vi "final.vi"() -> ()   [LabVIEW 2020]
uses:
  <vilib>/Simulation/Scripting/Companion Diagram/SimConfigNode/SimParams.ctl
  <vilib>/Simulation/Scripting/Companion Diagram/SimConfigNode/_simSolvers.ctl
  <vilib>/Simulation/Implementation/Shared/SIMSCR Execution Mode.ctl
  <vilib>/Simulation/Param Hierarchy/Typedefs/SIMPH Param Control Actions.ctl
  <vilib>/Simulation/Implementation/Shared/SIM limit type.ctl
  <vilib>/Simulation/Implementation/Shared/NILVSim_ParamChanged.vi
  <vilib>/Simulation/Implementation/Shared/NILVSIM_BeginStep.vi
  <vilib>/Simulation/SignalArithmetic/Implementation/NILVSim Gain.llb/SIM Gain (scalar).vi
  <vilib>/Simulation/ContinuousLinear/Implementation/NILVSim Derivative.llb/SIM derivative (scalar).vi
  <vilib>/Simulation/SignalDisplay/Implementation/NILVSim Time Waveform.llb/SIM Time Waveform (vector).vi
  <vilib>/Simulation/ContinuousLinear/Implementation/NILVSim Integrator new.llb/SIM Integrator distributor (scalar).vi
  <vilib>/Simulation/ContinuousLinear/Implementation/NILVSim Integrator new.llb/SIM Integrator collector (scalar).vi
  <vilib>/Simulation/SignalDisplay/Implementation/NILVSim Time Waveform.llb/SIM Time Waveform (scalar).vi
  <vilib>/Simulation/Implementation/Shared/SIM Is Init or Final Stage.vi
  <vilib>/Simulation/Implementation/Shared/NILVSim_Manager.vi
  <vilib>/Utility/error.llb/Clear Errors.vi
  <vilib>/Simulation/Implementation/Shared/NILVSim_FinalizeModel.vi
  <vilib>/imath/engines/lvmath2/RunTimeEngine/Managers/WorkSpace/UID Generator.vi
  <vilib>/imath/engines/lvmath2/RunTimeEngine/RunTimeType/NIMS_RunTimeType_From StrictType (excl LVString).vi
  <instcachedir>/0/NIMS_RunTimeType_From StrictType (excl LVString)_283B1B2000484AAA8744D21CE97EA49F.lvgen/NIMS_RunTimeType_From StrictType (excl LVString)_283B1B2000484AAA8744D21CE97EA49F_000.vi
  <vilib>/imath/engines/lvmath2/RunTimeEngine/LocalVariableDefStatement/MC_LocalVariableDefStatement_Display.vi
  <vilib>/imath/engines/lvmath/Plug In/Control Design/BuiltInFunctions/tf/NIMS_CD_tf(num,den,Ts).vi
  <instcachedir>/0/NIMS_RunTimeType_From StrictType (excl LVString)_283B1B2000484AAA8744D21CE97EA49F.lvgen/NIMS_RunTimeType_From StrictType (excl LVString)_283B1B2000484AAA8744D21CE97EA49F_031.vi
  <vilib>/imath/engines/lvmath/Plug In/Control Design/BuiltInFunctions/series/NIMS_CD_series(TF,TF).vi
  <vilib>/imath/engines/lvmath/Plug In/Control Design/BuiltInFunctions/feedback/NIMS_CD_feedback(TF,K,SIGN).vi
  <vilib>/imath/engines/lvmath/Plug In/Control Design/BuiltInFunctions/poles/NIMS_CD_poles(TF).vi
  <vilib>/imath/engines/lvmath2/RunTimeEngine/Managers/SymbolTable/Clear UID.vi
  <vilib>/imath/engines/lvmath2/RunTimeEngine/NodeEndStatement/NIMS_NodeEndStatement_Output.vi
  <instcachedir>/0/NIMS_NodeEndStatement_Output_53EC0D466D134D7ABD903AC30B43404B.lvgen/NIMS_NodeEndStatement_Output_53EC0D466D134D7ABD903AC30B43404B_000.vi
  <instcachedir>/0/NIMS_NodeEndStatement_Output_53EC0D466D134D7ABD903AC30B43404B.lvgen/NIMS_NodeEndStatement_Output_53EC0D466D134D7ABD903AC30B43404B_010.vi
  <vilib>/imath/engines/lvmath2/RunTimeEngine/ErrorHandling/NIMS_Finalize Error.vi
  <vilib>/addons/Control Design/_Utility/Model Viewer.llb/Model Viewer SubVI/cd_Draw Transfer Function Equation (TF).vi
  <vilib>/Simulation/Implementation/Shared/SIM Unbundle Sim Info.vi
  <vilib>/Simulation/Implementation/Shared/NILVSim_Initialize.vi
  <vilib>/Simulation/Utility/Implementation/NILVSim Get Time and IsAcceptedStep.vi
  <vilib>/Platform/system.llb/Beep.vi
  <vilib>/Simulation/Implementation/Shared/SIMSH Read Queue.vi
  <vilib>/Simulation/Implementation/Shared/NILVSim_GetModelError.vi
  <vilib>/Simulation/Implementation/Shared/SIM Bundle Sim Info.vi
  <vilib>/Simulation/Scripting/Companion Diagram/SimConfigNode/SimDog.xnode
  <vilib>/Simulation/Implementation/XNodeFramework/SimXNode/SimX.xnode
  <vilib>/Simulation/ContinuousLinear/Implementation/NILVSim Integrator new.llb/SIM Integrator (scalar).vi
  <vilib>/addons/Control Design/_Utility/NI_CD_Model Viewer.lvlib
  <vilib>/imath/engines/lvmath2/RunTimeEngine/Managers/SymbolTable/NIMS_WorkSpace.lvlib
  <vilib>/Simulation/Implementation/Shared/NI_SIM_Implementation.lvlib
panel:
  out "Pososto sfalmatos peiramatikhs apo thewrtikh%":dbl format="%#_3g"
  out "Torque":waveform(dbl)(graph)
  out "Live gwniakh ta/xta":dynamicdata(graph)
  out "Gnwiakh ta/xta live":dbl
  out "Vout live":dbl
  out "p":cdb[](array[numeric])
  out "Gclosed with PID":picture
  out "PID open":picture
  out "Vout":dbl
  out "Current":dbl
  out "Gwniakh tax/ta":dbl
  in  "Vin":dbl
  out "Vout/Vin":waveform(dbl)[](graph)
  in  "Ki":dbl
  in  "Kd":dbl
  in  "Kp":dbl
  in  "R":dbl
  in  "b":dbl
  in  "L":dbl
  in  "J":dbl
  in  "K":dbl
  out "Gopen-DC Motor":picture
  out "Гщнйбкз фбч/фб":waveform(dbl)(graph)
  out "Current":waveform(dbl)(graph)
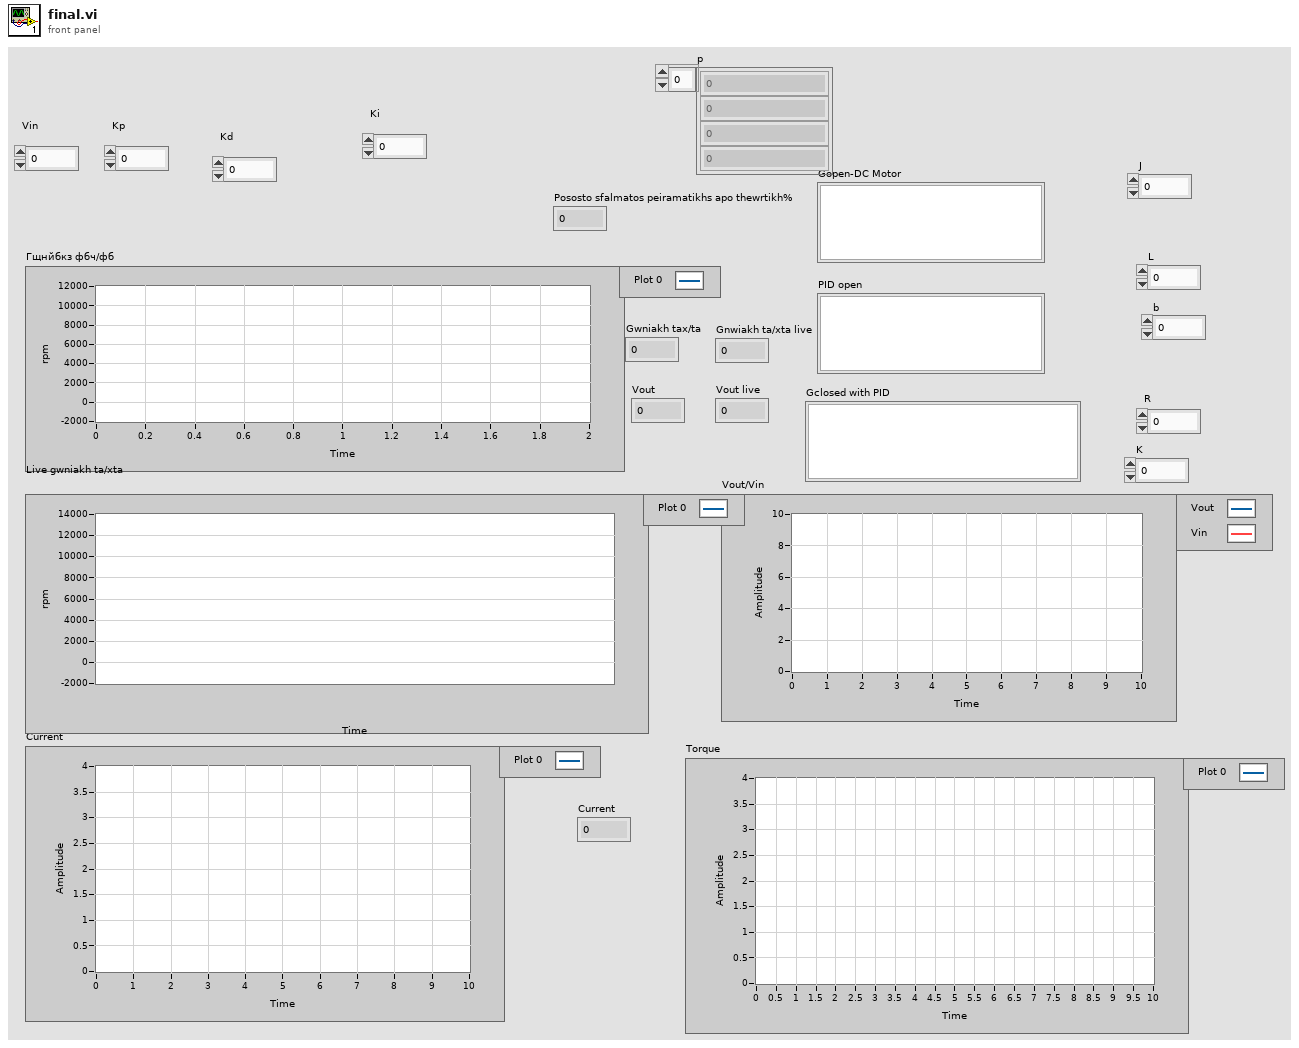
[diagram p1: front panel]
types:
  T1 = typedef "NI_LinSys_Model Typedefs.lvlib/CD Transfer Function Model (MIMO).ctl" = cluster{"properties":T2, "transfer function(s)":T3[][]}
  T2 = typedef "NI_LinSys_Model Typedefs.lvlib/CD General Elements.ctl" = cluster{"Model name":string, "Input names":string[], "Output names":string[], "Input Delays":dbl[], "Output Delays":dbl[], "Sampling Time":dbl, "Notes":string}
  T3 = typedef "NI_LinSys_Model Typedefs.lvlib/CD Transfer Function Model (SISO).ctl" = cluster{"Numerator":dbl[], "Denominator":dbl[], "delay":dbl}
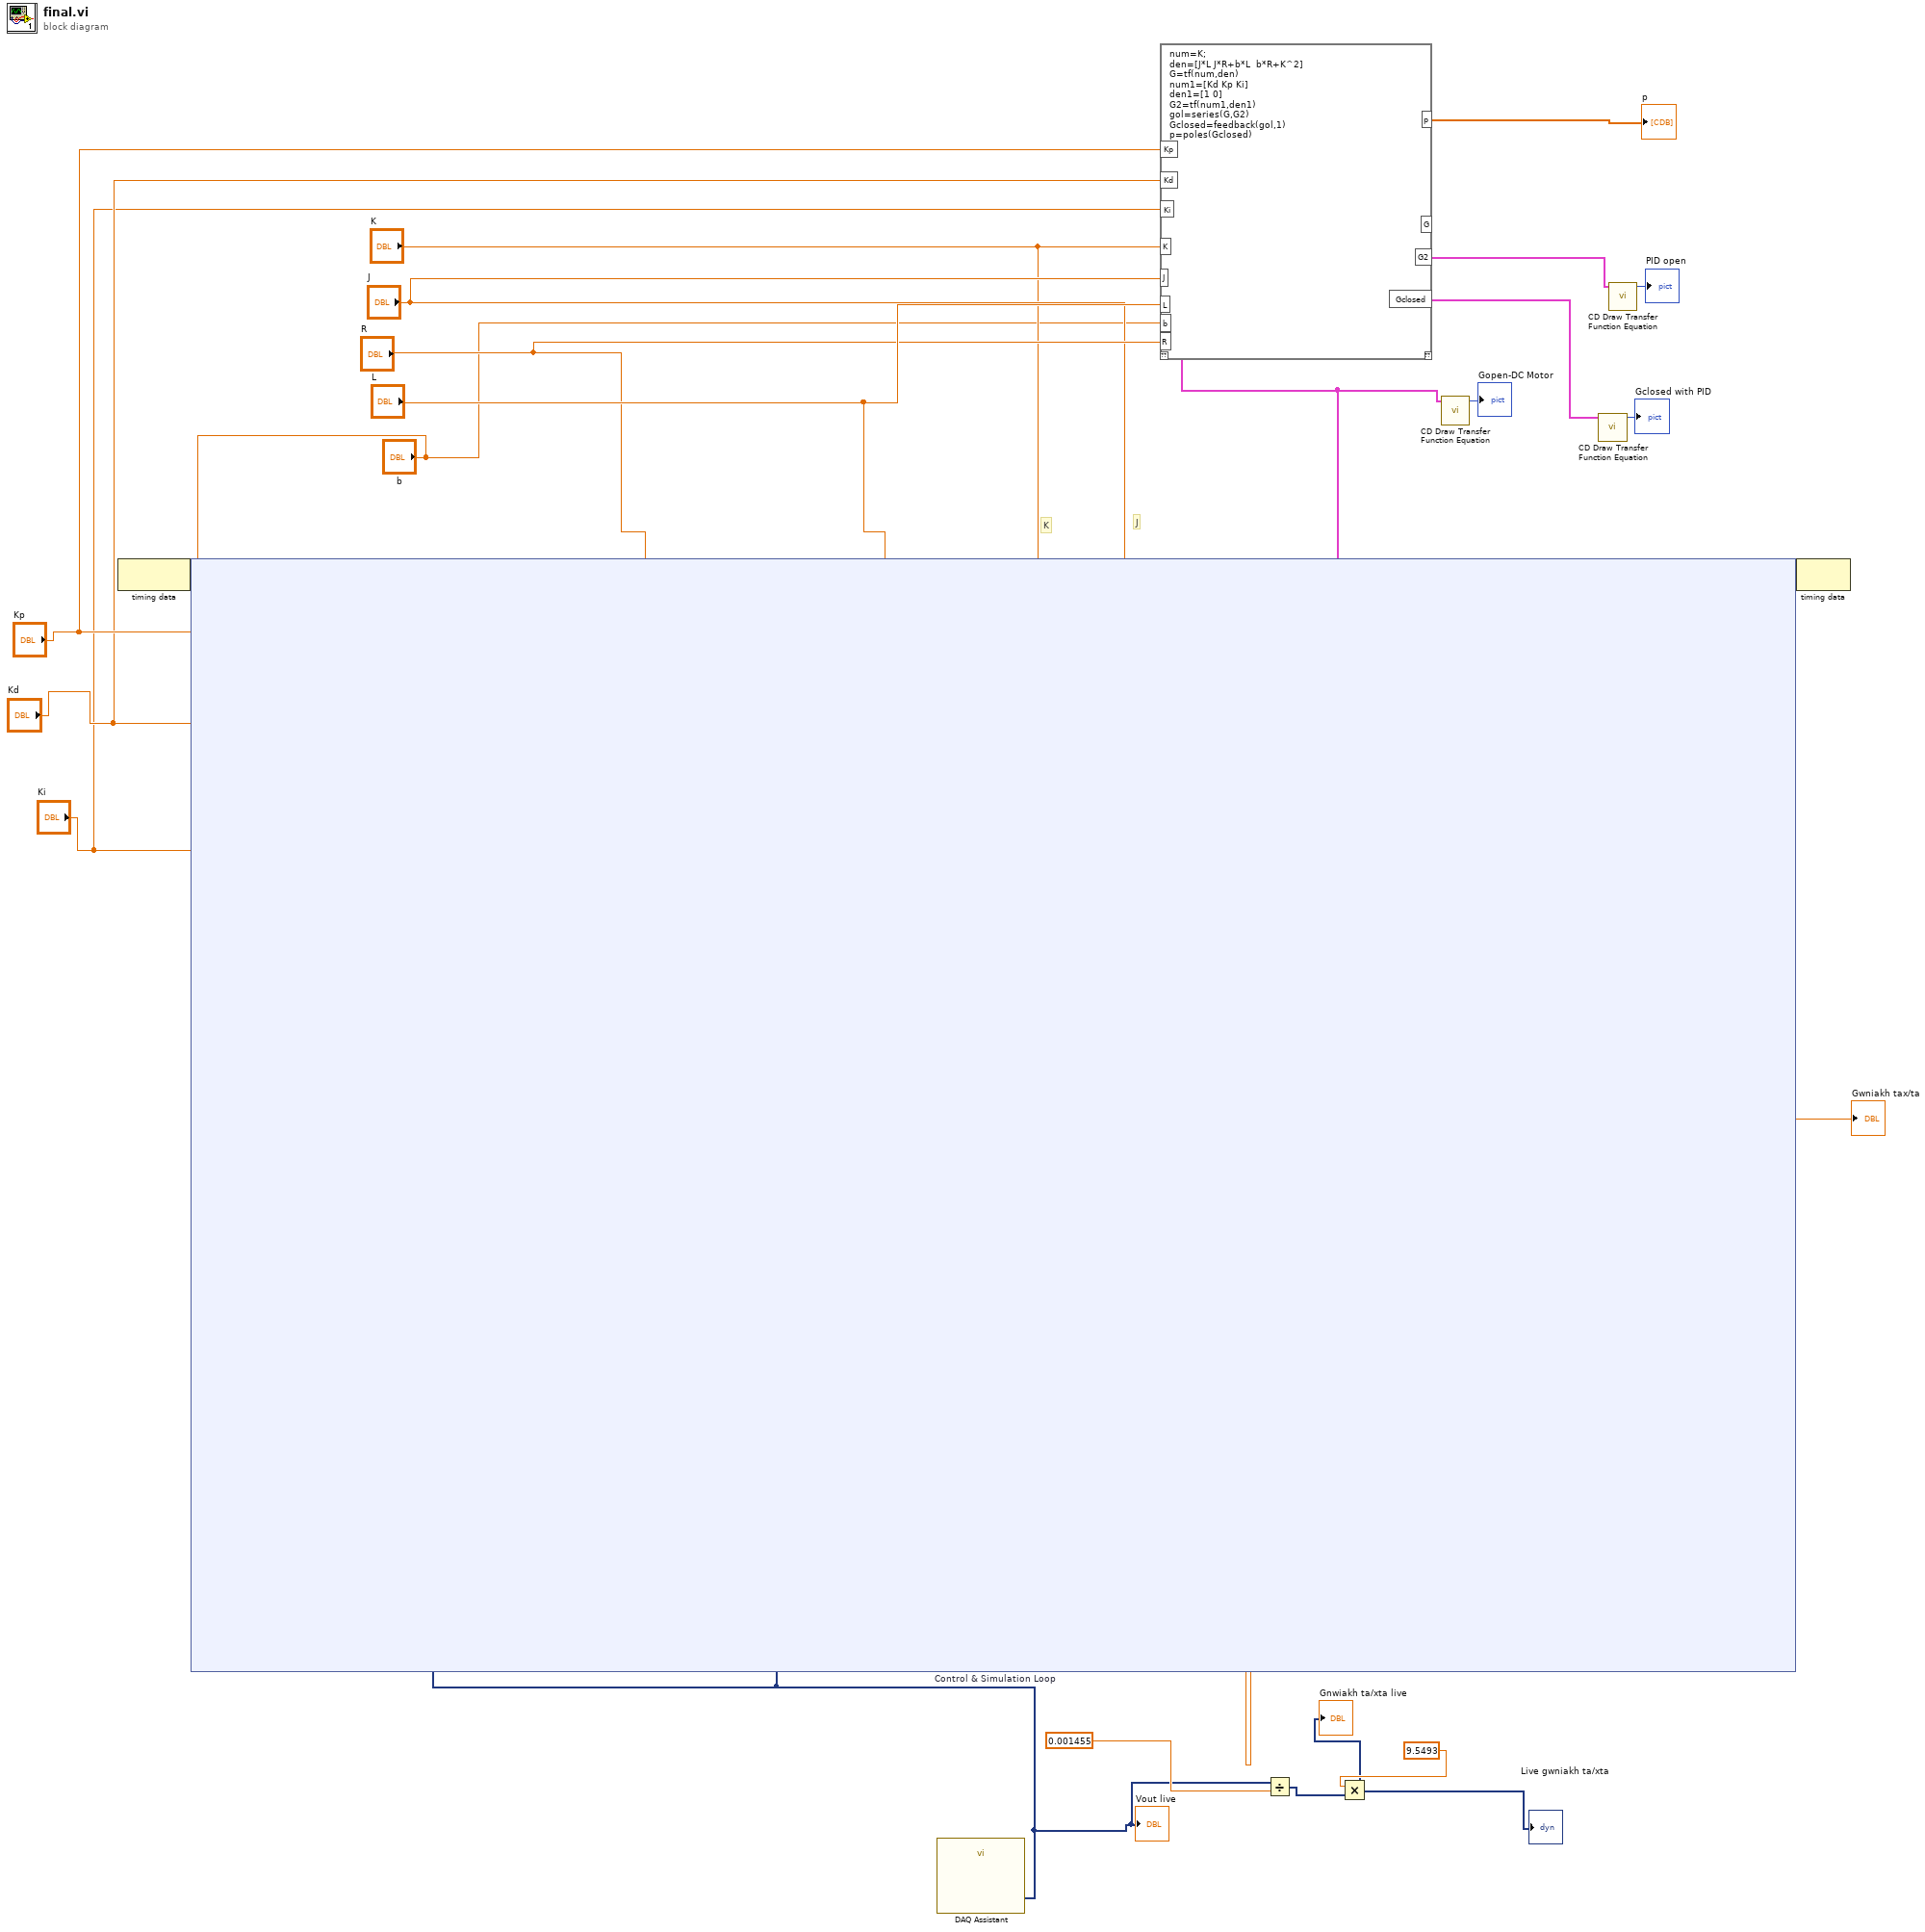
[diagram p0: block diagram]
diagram:
  # "J"
  # "K"
  n1 = node-c288() -> (w23:variant)  [unwired: 1 in]
  n2 = call "DAQ Assistant"() -> ("data"=w1:dynamicdata)  [unwired: 17 in, 2 out]
  "Vout live" <- w1
  n3 = mathscript code="num=K;\nden=[J*L J*R+b*L  b*R+K^2]\nG=tf(num,den)\nnum1=[Kd Kp Ki]\nden1=[1 0]\nG2=tf(num1,den1)\ngol=series(G,G2)\nGclosed=feedback(gol,1)\np=poles(Gclosed)"("K"="K", "J"="J", "L"="L", "b"="b", "R"="R", "Kp"="Kp", "Kd"="Kd", "Ki"="Ki") -> ("G"=w20:T1, "G2"=w10:T1, "Gclosed"=w8:T1, "p"=→"p":cdb[])  [unwired: 1 in, 1 out]
  n4 = node-c254 "Control & Simulation Loop"(w23, w20, "L", "R", "J", "K", "Ki", "Kd", "Kp", "b", w1, w1) -> (w22:variant, →"Gwniakh tax/ta":dbl)
  n5 = Divide(x=w1, y=0.001455 ("Operand1 2")) -> (x/y=w3:dynamicdata)
  n6 = Multiply(x=9.5493 ("Operand1 2"), y=w3) -> (x*y=→"Gnwiakh ta/xta live" →"Live gwniakh ta/xta":dynamicdata)
  n7 = call-poly <vilib>:"CD Draw Transfer Function Equation.vi"("Transfer Function Model"=w20) -> ("Equation"=→"Gopen-DC Motor":picture)  [unwired: 8 in, 2 out]
  n8 = call-poly <vilib>:"CD Draw Transfer Function Equation.vi"("Transfer Function Model"=w8) -> ("Equation"=→"Gclosed with PID":picture)  [unwired: 8 in, 2 out]
  n9 = call-poly <vilib>:"CD Draw Transfer Function Equation.vi"("Transfer Function Model"=w10) -> ("Equation"=→"PID open":picture)  [unwired: 8 in, 2 out]
  n10 = node-c288(w22) -> ()  [unwired: 1 out]
